vi "TempConversion.vi"() -> ()   [LabVIEW 2017]
panel:
  in  "Case Value":i32
  out "size(s)":i32
  out "element":dbl
  in  "index":i32
  out "Array 4":bool[](array[boolean])
  in  "Array 3":bool[](array[boolean])
  out "Array 2":dbl[](array[slide]) scale=0.0..10.0
  in  "Array":dbl[](array[numeric])
  out "Waveform Graph":dbl[](graph)
  out "Temperature Value (C)":dbl
  out "Waveform Chart":dbl(graph)
  in  "stop":bool
  in  "Temperature (F)":dbl(slide) scale=0.0..200.0
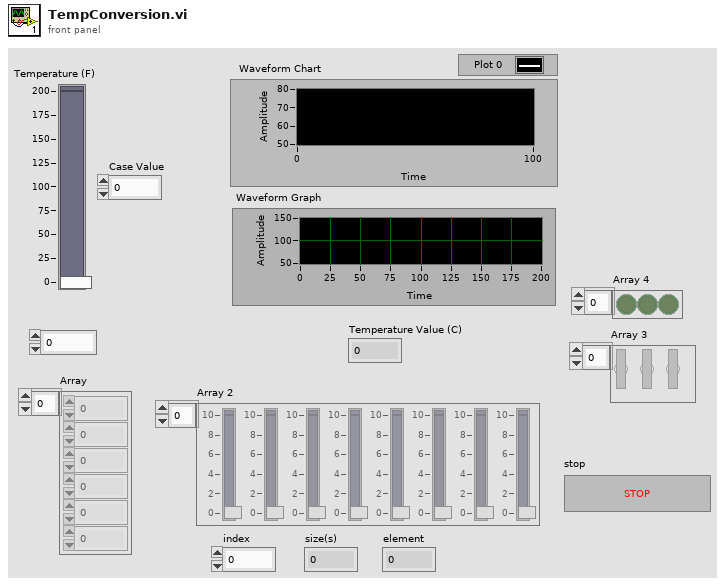
[diagram p1: front panel]
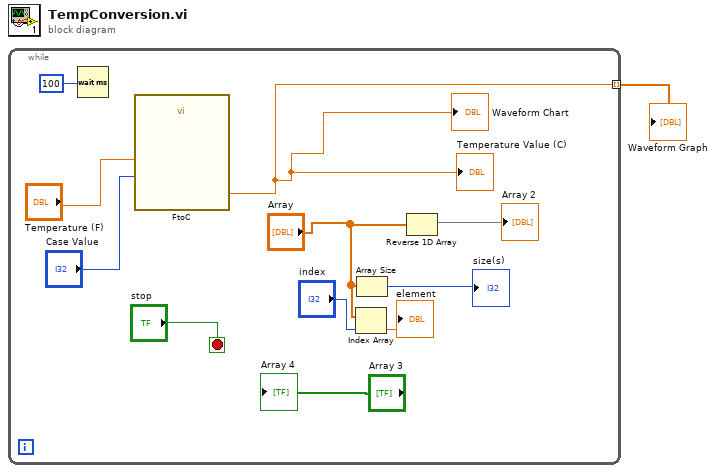
[diagram p0: block diagram]
diagram:
  n1 = while {
    tunnel: [w3] -> w1 mode=indexing
    stop <- "stop" stop-if-true
    n2 = Wait (ms)(milliseconds to wait=100) -> ()  [unwired: 1 out]
    n3 = call "FtoC.vi"("Temperature (F)"="Temperature (F)", "Case Value"="Case Value") -> ("Numeric"=w3:dbl)
    "Waveform Chart" <- w3
    "Temperature Value (C)" <- w3
    n4 = Index Array(array="Array", index="index") -> (element=→"element":dbl)
    n5 = Array Size(array="Array") -> (size(s)=→"size(s)":i32)
    n6 = Reverse 1D Array(array="Array") -> (reversed array=→"Array 2":dbl[])
    "Array 4" <- "Array 3"
  }
  "Waveform Graph" <- w1
